vi "ResetGyroOnTurn.vi"(0 "Drive Train Metrics in":T1) -> (7 "Drive Train Metrics Out":T1)   [LabVIEW 2014]
uses:
  Drive Train Metrics.ctl
  CmdFlag.ctl
  DriveTrainCals.vi
  DriveCals.vi
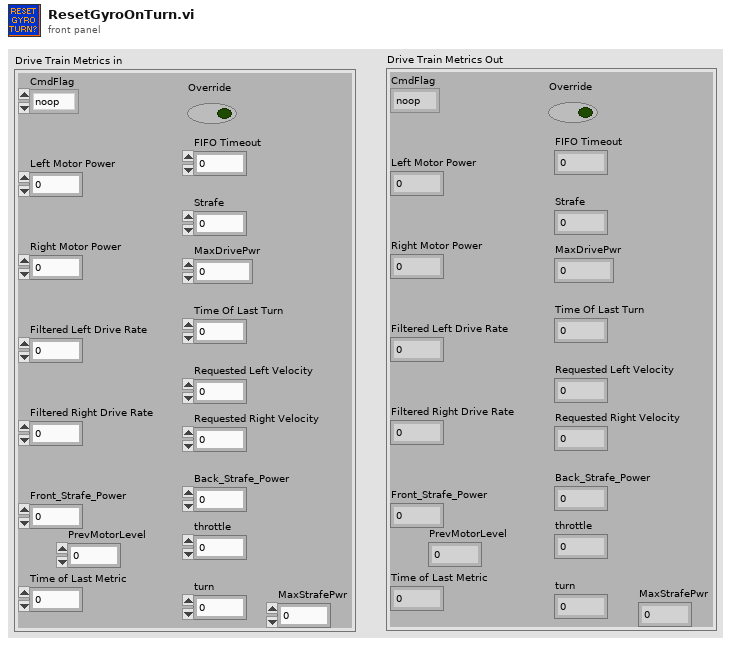
[diagram p1: front panel]
types:
  T1 = typedef "Drive Train Metrics.ctl" = cluster{"CmdFlag":T2, "Right Motor Power":dbl, "Left Motor Power":dbl, "Filtered Left Drive Rate":dbl, "Filtered Right Drive Rate":dbl, "Time of Last Metric":u32, "FIFO Timeout":i32, "Requested Left Velocity":dbl, "Requested Right Velocity":dbl, "throttle":dbl, "turn":dbl, "MaxDrivePwr":dbl, "Strafe":dbl, "Override":bool, "Time Of Last Turn":dbl, "Front_Strafe_Power":dbl, "Back_Strafe_Power":dbl, "MaxStrafePwr":dbl, "PrevMotorLevel":u8}
  T2 = typedef "CmdFlag.ctl" = enum16{"noop", "logflag", "suspend", "resume"}
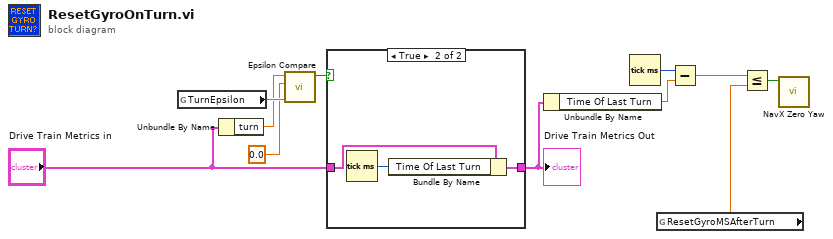
[diagram p0: block diagram]
diagram:
  n1 = global read "DriveTrainCals.vi" "TurnEpsilon"() -> (w11:dbl)
  n2 = Unbundle By Name("Drive Train Metrics in") -> ("turn"=w2:dbl)
  n3 = call "Epsilon Compare.vi"("Epsilon"=w11, "Value2"=0.0, "Value1"=w2) -> ("Boolean"=w5:bool)  [unwired: 8 in]
  n4 = case shown="True" w5 {
    tunnel: "Drive Train Metrics in" -> [w12 w15]
    tunnel: [w12 w13] -> w10
    frame False {
    }
    frame True {
      n5 = Tick Count (ms)() -> (millisecond timer value=w14:u32)
      n6 = Bundle By Name(cluster=w15, "Time Of Last Turn"=w14) -> (w13:T1)
    }
  }
  "Drive Train Metrics Out" <- w10
  n7 = Unbundle By Name(w10) -> ("Time Of Last Turn"=w7:dbl)
  n8 = Tick Count (ms)() -> (millisecond timer value=w8:u32)
  n9 = global read "DriveCals.vi" "ResetGyroMSAfterTurn"() -> (w1:dbl)
  n10 = Subtract(x=w8, y=w7) -> (x-y=w6:dbl)
  n11 = Less Or Equal?(x=w6, y=w1) -> (x <= y?=w9:bool)
  n12 = call "NavX Zero Yaw.vi"("Reset NavX Yaw"=w9) -> ()  [unwired: 11 in]
